vi "Control Cylinders.vi"(8 "error in (no error)":errorcluster, 9 "Cylinder 2":bool, 10 "Cylinder 1":bool, 11 "Process Settings in":refnum<class "Process Settings.lvclass">) -> (0 "error out":errorcluster, 3 "Process Settings out":refnum<class "Process Settings.lvclass">)   [LabVIEW 2017, in "Expansion.lvclass"]
uses:
  Expansion.lvclass
  Process Settings/Process Settings.lvclass
  Hardware Settings/Type Defs/Hardware Types.ctl
  Process Settings/Process Settings.lvclass/Process Settings.ctl
  Process Settings/Accessors/Read Hardware Settings.vi
  Hardware Settings/Hardware Settings.lvclass
  Hardware Settings/Hardware Types/Generic/Generic Hardware.lvclass
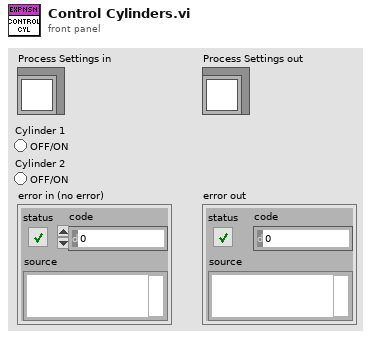
[diagram p1: front panel]
types:
  T1 = typedef "Hardware Settings.lvclass/Hardware Types.ctl" = enum16{"Tank Chamber Pressure and Temperature", "Tank Valve Controls", "Motor On/Off and Direction Control", "Limit Switches", "IR Temperature", "Pneumatic Cylinder Actuation", "Expansion Temperature Setpoint"}
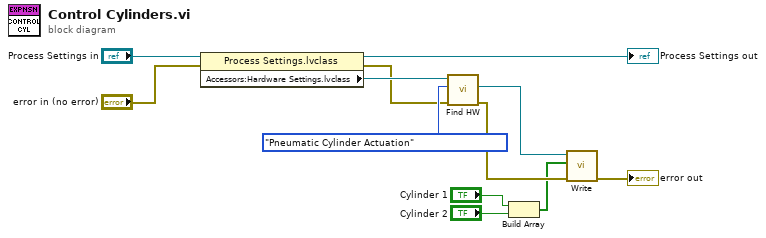
[diagram p0: block diagram]
diagram:
  n1 = property class="Process Settings.lvclass"(reference="Process Settings in", error in="error in (no error)") -> (reference out=→"Process Settings out":refnum<class "Process Settings.lvclass">, error out=w1:errorcluster, "Accessors:Hardware Settings.lvclass"=w5:refnum<class "Hardware Settings.lvclass">)
  n2 = call "Find HW.vi"("error in (no error)"=w1, "HW Item"=Hardware_Types."Pneumatic Cylinder Actuation", "Hardware Settings in"=w5) -> ("error out"=w11:errorcluster, "Selected Hardware Out"=w10:refnum<class "Generic Hardware.lvclass">)  [unwired: 6 in, 1 out]
  n3 = Build Array("Cylinder 1", "Cylinder 2") -> (w6:bool[])
  n4 = call-dynamic "Write.vi"("error in (no error)"=w11, "Input"=w6, "Generic Hardware in"=w10) -> ("error out"=→"error out":errorcluster)  [unwired: 7 in, 1 out]
